vi "メイン.vi"() -> (2 "測定周期/ms":dbl, 3 "値転記用配列":T2[](array[typedef]))   [LabVIEW 2021] (continued)
                          n3920 = Add(x=6, y=w6513) -> (x+y=w6506:i32)
                          n3921 = Add(x=w6513, y=7) -> (x+y=w6504:i32)
                          n3922 = local read "csv作成表"() -> (w6500:string[][])
                          n3923 = Unbundle By Name(w6511) -> ("実測値(MAX)"=w6507:string, "実測値(MIN)"=w6508:string)
                          n3924 = Replace Array Subset(array=w6500, new element #1=w6507, index (row) #1=w6505, index (col) #1=w6506, new element #2=w6508, index (row) #2=w6505, index (col) #2=w6504) -> (w6502:string[][])
                          n3925 = Select(t=w6502, s=w6512, f=w6500) -> (s? t:f=w6503:string[][])
                          n3926 = local write "csv作成表"(w6503) -> ()
                        }
                        frame 5 {
                          w6523 = 2
                          # "B"
                          # "A"
                          # "csv作成の為表へクラスタ(実測値)書き込み"
                          # "⑤"
                          # "③"
                          # "④"
                          n3927 = local read "メインON/OFF_\n設定 6"() -> (w6534:T1)
                          n3928 = Unbundle By Name(w6534) -> ("使用ON/OFF"=w6530:bool)
                          n3929 = control-ref of="前回値転記用配列"() -> (w6528:refnum<vi>)
                          n3930 = local read "メイン設定_設定 6"() -> (w6535:T2)
                          n3931 = call "メイン_測定値配列_CSV転記サブ.vi"("メイン設定_設定入力"=w6535, "ループ反復数値入力"=w6532, "実測設定項目"=w6533, "使用ON/OFF"=w6530, "前回値転記用配列"=w6528) -> ("ループ反復数値出力"=w6531:i32, "メイン設定_設定出力"=w6529:T2)  [unwired: 5 in]
                          n3932 = local write "メイン設定_設定 6"(w6529) -> ()
                          n3933 = Add(x=7, y=w6531) -> (x+y=w6524:i32)
                          n3934 = Add(x=w6531, y=8) -> (x+y=w6522:i32)
                          n3935 = local read "csv作成表"() -> (w6518:string[][])
                          n3936 = Unbundle By Name(w6529) -> ("実測値(MAX)"=w6525:string, "実測値(MIN)"=w6526:string)
                          n3937 = Replace Array Subset(array=w6518, new element #1=w6525, index (row) #1=w6523, index (col) #1=w6524, new element #2=w6526, index (row) #2=w6523, index (col) #2=w6522) -> (w6520:string[][])
                          n3938 = Select(t=w6520, s=w6530, f=w6518) -> (s? t:f=w6521:string[][])
                          n3939 = local write "csv作成表"(w6521) -> ()
                        }
                        frame 6 {
                          w6541 = 2
                          # "B"
                          # "A"
                          # "csv作成の為表へクラスタ(実測値)書き込み"
                          # "⑤"
                          # "③"
                          # "④"
                          n3940 = local read "メインON/OFF_\n設定 7"() -> (w6552:T1)
                          n3941 = Unbundle By Name(w6552) -> ("使用ON/OFF"=w6548:bool)
                          n3942 = control-ref of="前回値転記用配列"() -> (w6546:refnum<vi>)
                          n3943 = local read "メイン設定_設定 7"() -> (w6553:T2)
                          n3944 = call "メイン_測定値配列_CSV転記サブ.vi"("メイン設定_設定入力"=w6553, "ループ反復数値入力"=w6550, "実測設定項目"=w6551, "使用ON/OFF"=w6548, "前回値転記用配列"=w6546) -> ("ループ反復数値出力"=w6549:i32, "メイン設定_設定出力"=w6547:T2)  [unwired: 5 in]
                          n3945 = local write "メイン設定_設定 7"(w6547) -> ()
                          n3946 = Add(x=8, y=w6549) -> (x+y=w6542:i32)
                          n3947 = Add(x=w6549, y=9) -> (x+y=w6540:i32)
                          n3948 = local read "csv作成表"() -> (w6536:string[][])
                          n3949 = Unbundle By Name(w6547) -> ("実測値(MAX)"=w6543:string, "実測値(MIN)"=w6544:string)
                          n3950 = Replace Array Subset(array=w6536, new element #1=w6543, index (row) #1=w6541, index (col) #1=w6542, new element #2=w6544, index (row) #2=w6541, index (col) #2=w6540) -> (w6538:string[][])
                          n3951 = Select(t=w6538, s=w6548, f=w6536) -> (s? t:f=w6539:string[][])
                          n3952 = local write "csv作成表"(w6539) -> ()
                        }
                        frame 7 {
                          w6559 = 2
                          # "B"
                          # "A"
                          # "csv作成の為表へクラスタ(実測値)書き込み"
                          # "⑤"
                          # "③"
                          # "④"
                          n3953 = local read "メインON/OFF_\n設定 8"() -> (w6570:T1)
                          n3954 = Unbundle By Name(w6570) -> ("使用ON/OFF"=w6566:bool)
                          n3955 = control-ref of="前回値転記用配列"() -> (w6564:refnum<vi>)
                          n3956 = local read "メイン設定_設定 8"() -> (w6571:T2)
                          n3957 = call "メイン_測定値配列_CSV転記サブ.vi"("メイン設定_設定入力"=w6571, "ループ反復数値入力"=w6568, "実測設定項目"=w6569, "使用ON/OFF"=w6566, "前回値転記用配列"=w6564) -> ("ループ反復数値出力"=w6567:i32, "メイン設定_設定出力"=w6565:T2)  [unwired: 5 in]
                          n3958 = local write "メイン設定_設定 8"(w6565) -> ()
                          n3959 = Add(x=9, y=w6567) -> (x+y=w6560:i32)
                          n3960 = Add(x=w6567, y=10) -> (x+y=w6558:i32)
                          n3961 = local read "csv作成表"() -> (w6554:string[][])
                          n3962 = Unbundle By Name(w6565) -> ("実測値(MAX)"=w6561:string, "実測値(MIN)"=w6562:string)
                          n3963 = Replace Array Subset(array=w6554, new element #1=w6561, index (row) #1=w6559, index (col) #1=w6560, new element #2=w6562, index (row) #2=w6559, index (col) #2=w6558) -> (w6556:string[][])
                          n3964 = Select(t=w6556, s=w6566, f=w6554) -> (s? t:f=w6557:string[][])
                          n3965 = local write "csv作成表"(w6557) -> ()
                        }
                        frame 8 {
                          w6577 = 2
                          # "B"
                          # "A"
                          # "csv作成の為表へクラスタ(実測値)書き込み"
                          # "⑤"
                          # "③"
                          # "④"
                          n3966 = local read "メインON/OFF_\n設定 9"() -> (w6588:T1)
                          n3967 = Unbundle By Name(w6588) -> ("使用ON/OFF"=w6584:bool)
                          n3968 = control-ref of="前回値転記用配列"() -> (w6582:refnum<vi>)
                          n3969 = local read "メイン設定_設定 9"() -> (w6589:T2)
                          n3970 = call "メイン_測定値配列_CSV転記サブ.vi"("メイン設定_設定入力"=w6589, "ループ反復数値入力"=w6586, "実測設定項目"=w6587, "使用ON/OFF"=w6584, "前回値転記用配列"=w6582) -> ("ループ反復数値出力"=w6585:i32, "メイン設定_設定出力"=w6583:T2)  [unwired: 5 in]
                          n3971 = local write "メイン設定_設定 9"(w6583) -> ()
                          n3972 = Add(x=10, y=w6585) -> (x+y=w6578:i32)
                          n3973 = Add(x=w6585, y=11) -> (x+y=w6576:i32)
                          n3974 = local read "csv作成表"() -> (w6572:string[][])
                          n3975 = Unbundle By Name(w6583) -> ("実測値(MAX)"=w6579:string, "実測値(MIN)"=w6580:string)
                          n3976 = Replace Array Subset(array=w6572, new element #1=w6579, index (row) #1=w6577, index (col) #1=w6578, new element #2=w6580, index (row) #2=w6577, index (col) #2=w6576) -> (w6574:string[][])
                          n3977 = Select(t=w6574, s=w6584, f=w6572) -> (s? t:f=w6575:string[][])
                          n3978 = local write "csv作成表"(w6575) -> ()
                        }
                        frame 9 {
                          w6595 = 2
                          # "B"
                          # "A"
                          # "csv作成の為表へクラスタ(実測値)書き込み"
                          # "⑤"
                          # "③"
                          # "④"
                          n3979 = local read "メインON/OFF_\n設定 10"() -> (w6606:T1)
                          n3980 = Unbundle By Name(w6606) -> ("使用ON/OFF"=w6602:bool)
                          n3981 = control-ref of="前回値転記用配列"() -> (w6600:refnum<vi>)
                          n3982 = local read "メイン設定_設定 10"() -> (w6607:T2)
                          n3983 = call "メイン_測定値配列_CSV転記サブ.vi"("メイン設定_設定入力"=w6607, "ループ反復数値入力"=w6604, "実測設定項目"=w6605, "使用ON/OFF"=w6602, "前回値転記用配列"=w6600) -> ("ループ反復数値出力"=w6603:i32, "メイン設定_設定出力"=w6601:T2)  [unwired: 5 in]
                          n3984 = local write "メイン設定_設定 10"(w6601) -> ()
                          n3985 = Add(x=11, y=w6603) -> (x+y=w6596:i32)
                          n3986 = Add(x=w6603, y=12) -> (x+y=w6594:i32)
                          n3987 = local read "csv作成表"() -> (w6590:string[][])
                          n3988 = Unbundle By Name(w6601) -> ("実測値(MAX)"=w6597:string, "実測値(MIN)"=w6598:string)
                          n3989 = Replace Array Subset(array=w6590, new element #1=w6597, index (row) #1=w6595, index (col) #1=w6596, new element #2=w6598, index (row) #2=w6595, index (col) #2=w6594) -> (w6592:string[][])
                          n3990 = Select(t=w6592, s=w6602, f=w6590) -> (s? t:f=w6593:string[][])
                          n3991 = local write "csv作成表"(w6593) -> ()
                        }
                        frame 10 {
                          w6613 = 2
                          # "B"
                          # "A"
                          # "csv作成の為表へクラスタ(実測値)書き込み"
                          # "⑤"
                          # "③"
                          # "④"
                          n3992 = local read "メインON/OFF_\n設定 11"() -> (w6624:T1)
                          n3993 = Unbundle By Name(w6624) -> ("使用ON/OFF"=w6620:bool)
                          n3994 = control-ref of="前回値転記用配列"() -> (w6618:refnum<vi>)
                          n3995 = local read "メイン設定_設定 11"() -> (w6625:T2)
                          n3996 = call "メイン_測定値配列_CSV転記サブ.vi"("メイン設定_設定入力"=w6625, "ループ反復数値入力"=w6622, "実測設定項目"=w6623, "使用ON/OFF"=w6620, "前回値転記用配列"=w6618) -> ("ループ反復数値出力"=w6621:i32, "メイン設定_設定出力"=w6619:T2)  [unwired: 5 in]
                          n3997 = local write "メイン設定_設定 11"(w6619) -> ()
                          n3998 = Add(x=12, y=w6621) -> (x+y=w6614:i32)
                          n3999 = Add(x=w6621, y=13) -> (x+y=w6612:i32)
                          n4000 = local read "csv作成表"() -> (w6608:string[][])
                          n4001 = Unbundle By Name(w6619) -> ("実測値(MAX)"=w6615:string, "実測値(MIN)"=w6616:string)
                          n4002 = Replace Array Subset(array=w6608, new element #1=w6615, index (row) #1=w6613, index (col) #1=w6614, new element #2=w6616, index (row) #2=w6613, index (col) #2=w6612) -> (w6610:string[][])
                          n4003 = Select(t=w6610, s=w6620, f=w6608) -> (s? t:f=w6611:string[][])
                          n4004 = local write "csv作成表"(w6611) -> ()
                        }
                        frame 11 {
                          w6631 = 2
                          # "B"
                          # "A"
                          # "csv作成の為表へクラスタ(実測値)書き込み"
                          # "⑤"
                          # "③"
                          # "④"
                          n4005 = local read "メインON/OFF_\n設定 12"() -> (w6642:T1)
                          n4006 = Unbundle By Name(w6642) -> ("使用ON/OFF"=w6638:bool)
                          n4007 = control-ref of="前回値転記用配列"() -> (w6636:refnum<vi>)
                          n4008 = local read "メイン設定_設定 12"() -> (w6643:T2)
                          n4009 = call "メイン_測定値配列_CSV転記サブ.vi"("メイン設定_設定入力"=w6643, "ループ反復数値入力"=w6640, "実測設定項目"=w6641, "使用ON/OFF"=w6638, "前回値転記用配列"=w6636) -> ("ループ反復数値出力"=w6639:i32, "メイン設定_設定出力"=w6637:T2)  [unwired: 5 in]
                          n4010 = local write "メイン設定_設定 12"(w6637) -> ()
                          n4011 = Add(x=13, y=w6639) -> (x+y=w6632:i32)
                          n4012 = Add(x=w6639, y=14) -> (x+y=w6630:i32)
                          n4013 = local read "csv作成表"() -> (w6626:string[][])
                          n4014 = Unbundle By Name(w6637) -> ("実測値(MAX)"=w6633:string, "実測値(MIN)"=w6634:string)
                          n4015 = Replace Array Subset(array=w6626, new element #1=w6633, index (row) #1=w6631, index (col) #1=w6632, new element #2=w6634, index (row) #2=w6631, index (col) #2=w6630) -> (w6628:string[][])
                          n4016 = Select(t=w6628, s=w6638, f=w6626) -> (s? t:f=w6629:string[][])
                          n4017 = local write "csv作成表"(w6629) -> ()
                        }
                      }
                    }
                  }
                }
                n4018 = local write "値転記用配列"(w6400) -> ()
                n4019 = flat-sequence {
                  tunnel: [w6415] -> w6401
                  tunnel: w6400 -> [w6415]
                  frame #0 {
                    w6410 = T9 {"Horizontal"=-51, "Vertical"=792} ("座標 11")
                    n4020 = control-ref of="このVI"() -> (w6414:refnum<vi>)
                    n4021 = property on="ペーン 2" class="Pane"("Origin"=w6410) -> ()  [unwired: 2 in, 2 out]
                    n4022 = property on="ペーン 2" class="Pane"("Origin"=w6410) -> ()  [unwired: 2 in, 2 out]
                    n4023 = control-ref of="このVI"() -> (w6412:refnum<vi>)
                    n4024 = Unbundle(w6410) -> ("Vertical"=w6413:i16)  [unwired: 1 out]
                    n4025 = Unbundle(w6410) -> ("Vertical"=w6411:i16)  [unwired: 1 out]
                    n4026 = call "メイン_装飾移動サブ.vi"("Y軸座標入力"=w6413, "VI入力"=w6414) -> ()  [unwired: 10 in]
                    n4027 = call "メイン_装飾枠移動サブ.vi"("Y軸座標入力"=w6411, "VI入力"=w6412) -> ()  [unwired: 10 in]
                  }
                }
              }
              frame #1 {
                w6646 = T8."Enabled" ("無効")
                # "⑪ボタンの無効解除"
                n4028 = for {
                  N: 12 -> [_]
                  tunnel: w6646 -> [w6648]
                  i -> [w6649]
                  n4029 = case shown="11" w6649 {
                    tunnel: w6648 -> [w6650 w6651 w6652 w6653 w6654 w6655 w6656 w6657 w6658 w6659 w6660 w6661]
                    frame 0, Default {
                      n4030 = property on="メイン測定ボタン_単発 1" class="Bool (指定)"("DisabledEnum"=w6650) -> ()  [unwired: 2 in, 2 out]
                      n4031 = property on="メイン測定ボタン_連続 1" class="Bool (指定)"("DisabledEnum"=w6650) -> ()  [unwired: 2 in, 2 out]
                    }
                    frame 1 {
                      n4032 = property on="メイン測定ボタン_単発 2" class="Bool (指定)"("DisabledEnum"=w6651) -> ()  [unwired: 2 in, 2 out]
                      n4033 = property on="メイン測定ボタン_連続 2" class="Bool (指定)"("DisabledEnum"=w6651) -> ()  [unwired: 2 in, 2 out]
                    }
                    frame 2 {
                      n4034 = property on="メイン測定ボタン_単発 3" class="Bool (指定)"("DisabledEnum"=w6652) -> ()  [unwired: 2 in, 2 out]
                      n4035 = property on="メイン測定ボタン_連続 3" class="Bool (指定)"("DisabledEnum"=w6652) -> ()  [unwired: 2 in, 2 out]
                    }
                    frame 3 {
                      n4036 = property on="メイン測定ボタン_単発 4" class="Bool (指定)"("DisabledEnum"=w6653) -> ()  [unwired: 2 in, 2 out]
                      n4037 = property on="メイン測定ボタン_連続 4" class="Bool (指定)"("DisabledEnum"=w6653) -> ()  [unwired: 2 in, 2 out]
                    }
                    frame 4 {
                      n4038 = property on="メイン測定ボタン_単発 5" class="Bool (指定)"("DisabledEnum"=w6654) -> ()  [unwired: 2 in, 2 out]
                      n4039 = property on="メイン測定ボタン_連続 5" class="Bool (指定)"("DisabledEnum"=w6654) -> ()  [unwired: 2 in, 2 out]
                    }
                    frame 5 {
                      n4040 = property on="メイン測定ボタン_連続 6" class="Bool (指定)"("DisabledEnum"=w6655) -> ()  [unwired: 2 in, 2 out]
                      n4041 = property on="メイン測定ボタン_単発 6" class="Bool (指定)"("DisabledEnum"=w6655) -> ()  [unwired: 2 in, 2 out]
                    }
                    frame 6 {
                      n4042 = property on="メイン測定ボタン_連続 7" class="Bool (指定)"("DisabledEnum"=w6656) -> ()  [unwired: 2 in, 2 out]
                      n4043 = property on="メイン測定ボタン_単発 7" class="Bool (指定)"("DisabledEnum"=w6656) -> ()  [unwired: 2 in, 2 out]
                    }
                    frame 7 {
                      n4044 = property on="メイン測定ボタン_単発 8" class="Bool (指定)"("DisabledEnum"=w6657) -> ()  [unwired: 2 in, 2 out]
                      n4045 = property on="メイン測定ボタン_連続 8" class="Bool (指定)"("DisabledEnum"=w6657) -> ()  [unwired: 2 in, 2 out]
                    }
                    frame 8 {
                      n4046 = property on="メイン測定ボタン_単発 9" class="Bool (指定)"("DisabledEnum"=w6658) -> ()  [unwired: 2 in, 2 out]
                      n4047 = property on="メイン測定ボタン_連続 9" class="Bool (指定)"("DisabledEnum"=w6658) -> ()  [unwired: 2 in, 2 out]
                    }
                    frame 9 {
                      n4048 = property on="メイン測定ボタン_単発 10" class="Bool (指定)"("DisabledEnum"=w6659) -> ()  [unwired: 2 in, 2 out]
                      n4049 = property on="メイン測定ボタン_連続 10" class="Bool (指定)"("DisabledEnum"=w6659) -> ()  [unwired: 2 in, 2 out]
                    }
                    frame 10 {
                      n4050 = property on="メイン測定ボタン_単発 11" class="Bool (指定)"("DisabledEnum"=w6660) -> ()  [unwired: 2 in, 2 out]
                      n4051 = property on="メイン測定ボタン_連続 11" class="Bool (指定)"("DisabledEnum"=w6660) -> ()  [unwired: 2 in, 2 out]
                    }
                    frame 11 {
                      n4052 = property on="メイン測定ボタン_連続 12" class="Bool (指定)"("DisabledEnum"=w6661) -> ()  [unwired: 2 in, 2 out]
                      n4053 = property on="メイン測定ボタン_単発 12" class="Bool (指定)"("DisabledEnum"=w6661) -> ()  [unwired: 2 in, 2 out]
                    }
                  }
                }
                n4054 = local write "測定新値\nリセット用 12"(TRUE) -> ()
                n4055 = property on="TOPページへ" class="Bool"("DisabledEnum"=w6646) -> ()  [unwired: 2 in, 2 out]
                n4056 = property on="保存して終了" class="Bool"("DisabledEnum"=w6646) -> ()  [unwired: 2 in, 2 out]
                n4057 = property on="保存せずに" class="Bool"("DisabledEnum"=w6646) -> ()  [unwired: 2 in, 2 out]
              }
            }
          }
          frame True {
          }
        }
      }
    }
    n4058 = Wait (ms)(milliseconds to wait=10) -> ()  [unwired: 1 out]
  }
  n4059 = while {
    tunnel: w1 -> [w6668]
    tunnel: [w6667] -> w9
    shift-right: [w6664] -> w8
    shift-left: w2 -> [w6666]
    stop <- w6665 stop-if-true
    # "メインページのボタン操作時の動作"
    n4060 = event shown="[15] \"メイン測定ボタン_連続 1\": 値変更" {
      selector: _ -> [_ _ _ _ _ _ _ _ _ _ _ _ _ _ _ _ _ _ _ _ _ _ _ _ _ _ _ _ _ _ _ _ _ _ _ _ _ _ _ _ _ _ _ _ _ _ _ _ _ _ _]
      dyn-events: _ -> [_ _ _ _ _ _ _ _ _ _ _ _ _ _ _ _ _ _ _ _ _ _ _ _ _ _ _ _ _ _ _ _ _ _ _ _ _ _ _ _ _ _ _ _ _ _ _ _ _ _ _]
      timeout: _ -> [_ _ _ _ _ _ _ _ _ _ _ _ _ _ _ _ _ _ _ _ _ _ _ _ _ _ _ _ _ _ _ _ _ _ _ _ _ _ _ _ _ _ _ _ _ _ _ _ _ _ _]
      tunnel: w6668 -> [w6673 w6676 w6681 w6686 w6691 w6696 w6701 w6706 w6711 w6716 w6721 w6726 w6731 w6736 w6741 w6752 w6791 w6830 w6869 w6908 w6947 w6986 w7025 w7064 w7103 w7142 w7181 w7223 w7334 w7445 w7556 w7667 w7778 w7889 w8000 w8111 w8222 w8333 w8444 w8543 w8546 w8549 w8552 w8555 w8558 w8561 w8564 w8567 w8570 w8573 w8576]
      tunnel: [_ _ _ w6685 w6690 w6695 w6700 w6705 w6710 w6715 w6720 w6725 w6730 w6735 w6740 w6751 w6790 w6829 w6868 w6907 w6946 w6985 w7024 w7063 w7102 w7141 w7180 w7224 w7335 w7446 w7557 w7668 w7779 w7890 w8001 w8112 w8223 w8334 w8445 _ _ _ _ _ _ _ _ _ _ _ _] -> w6667
      tunnel: w6666 -> [w6671 w6674 w6680 w6683 w6688 w6693 w6698 w6703 w6708 w6713 w6718 w6723 w6728 w6733 w6738 w6749 w6788 w6827 w6866 w6905 w6944 w6983 w7022 w7061 w7100 w7139 w7178 w7221 w7332 w7443 w7554 w7665 w7776 w7887 w7998 w8109 w8220 w8331 w8442 w8542 w8545 w8548 w8551 w8554 w8557 w8560 w8563 w8566 w8569 w8572 w8575]
      tunnel: [w6672 w6675 w6678 w6684 w6689 w6694 w6699 w6704 w6709 w6714 w6719 w6724 w6729 w6734 w6739 w6750 w6789 w6828 w6867 w6906 w6945 w6984 w7023 w7062 w7101 w7140 w7179 w7222 w7333 w7444 w7555 w7666 w7777 w7888 w7999 w8110 w8221 w8332 w8443 _ _ _ _ _ _ _ _ _ _ _ _] -> w6664
      tunnel: [TRUE _ _ _ _ _ _ _ _ _ _ _ _ _ _ _ _ _ _ _ _ _ _ _ _ _ _ _ _ _ _ _ _ _ _ _ _ _ _ _ _ _ _ _ _ _ _ _ _ _ _] -> w6665
      tunnel: T8."Disabled" ("無効") -> [_ _ _ _ _ _ _ _ _ _ _ _ _ _ _ w6748 w6787 w6826 w6865 w6904 w6943 w6982 w7021 w7060 w7099 w7138 w7176 _ _ _ _ _ _ _ _ _ _ _ _ _ _ _ _ _ _ _ _ _ _ _ _]
      event "TOPページへ": Value Change {
        n4061 = event-data() -> ()  [unwired: 1 in, 6 out]
        n4062 = Enqueue Element(queue=w6673, element="TOPページへ", error in (no error)=w6671) -> (error out=w6672:errorcluster)  [unwired: 1 in, 2 out]
      }
      event "保存せずに": Value Change {
        # "メインページの保存せずに終了ボタンが押された時に動作"
        n4063 = event-data() -> ()  [unwired: 1 in, 1 out]
        n4064 = Enqueue Element(queue=w6676, element="保存せず", error in (no error)=w6674) -> (error out=w6675:errorcluster)  [unwired: 1 in, 2 out]
      }
      event "保存して終了": Value Change {
        n4065 = event-data() -> ()  [unwired: 1 in, 1 out]
        n4066 = Enqueue Element(queue=w6681, element="保存して終了", error in (no error)=w6680) -> (error out=w6678:errorcluster)  [unwired: 1 in, 2 out]
      }
      event Value Change {
        n4067 = event-data() -> ()  [unwired: 1 in, 6 out]
        n4068 = Enqueue Element(queue=w6686, element="値1クリア", error in (no error)=w6683) -> (queue out=w6685:refnum<queue>, error out=w6684:errorcluster)  [unwired: 1 in, 1 out]
      }
      event Value Change {
        # "①"
        # "複製時に変更する項目\n①キュー"
        n4069 = event-data() -> ()  [unwired: 1 in, 6 out]
        n4070 = Enqueue Element(queue=w6691, element="値2クリア", error in (no error)=w6688) -> (queue out=w6690:refnum<queue>, error out=w6689:errorcluster)  [unwired: 1 in, 1 out]
      }
      event Value Change {
        # "①"
        # "複製時に変更する項目\n①キュー"
        n4071 = event-data() -> ()  [unwired: 1 in, 6 out]
        n4072 = Enqueue Element(queue=w6696, element="値3クリア", error in (no error)=w6693) -> (queue out=w6695:refnum<queue>, error out=w6694:errorcluster)  [unwired: 1 in, 1 out]
      }
      event Value Change {
        # "①"
        # "複製時に変更する項目\n①キュー"
        n4073 = event-data() -> ()  [unwired: 1 in, 6 out]
        n4074 = Enqueue Element(queue=w6701, element="値4クリア", error in (no error)=w6698) -> (queue out=w6700:refnum<queue>, error out=w6699:errorcluster)  [unwired: 1 in, 1 out]
      }
      event Value Change {
        # "①"
        # "複製時に変更する項目\n①キュー"
        n4075 = event-data() -> ()  [unwired: 1 in, 6 out]
        n4076 = Enqueue Element(queue=w6706, element="値5クリア", error in (no error)=w6703) -> (queue out=w6705:refnum<queue>, error out=w6704:errorcluster)  [unwired: 1 in, 1 out]
      }
      event Value Change {
        # "①"
        # "複製時に変更する項目\n①キュー"
        n4077 = event-data() -> ()  [unwired: 1 in, 6 out]
        n4078 = Enqueue Element(queue=w6711, element="値6クリア", error in (no error)=w6708) -> (queue out=w6710:refnum<queue>, error out=w6709:errorcluster)  [unwired: 1 in, 1 out]
      }
      event Value Change {
        # "①"
        # "複製時に変更する項目\n①キュー"
        n4079 = event-data() -> ()  [unwired: 1 in, 6 out]
        n4080 = Enqueue Element(queue=w6716, element="値7クリア", error in (no error)=w6713) -> (queue out=w6715:refnum<queue>, error out=w6714:errorcluster)  [unwired: 1 in, 1 out]
      }
      event Value Change {
        # "①"
        # "複製時に変更する項目\n①キュー"
        n4081 = event-data() -> ()  [unwired: 1 in, 6 out]
        n4082 = Enqueue Element(queue=w6721, element="値8クリア", error in (no error)=w6718) -> (queue out=w6720:refnum<queue>, error out=w6719:errorcluster)  [unwired: 1 in, 1 out]
      }
      event Value Change {
        # "①"
        # "複製時に変更する項目\n①キュー"
        n4083 = event-data() -> ()  [unwired: 1 in, 6 out]
        n4084 = Enqueue Element(queue=w6726, element="値9クリア", error in (no error)=w6723) -> (queue out=w6725:refnum<queue>, error out=w6724:errorcluster)  [unwired: 1 in, 1 out]
      }
      event Value Change {
        # "①"
        # "複製時に変更する項目\n①キュー"
        n4085 = event-data() -> ()  [unwired: 1 in, 6 out]
        n4086 = Enqueue Element(queue=w6731, element="値10クリア", error in (no error)=w6728) -> (queue out=w6730:refnum<queue>, error out=w6729:errorcluster)  [unwired: 1 in, 1 out]
      }
      event Value Change {
        # "①"
        # "複製時に変更する項目\n①キュー"
        n4087 = event-data() -> ()  [unwired: 1 in, 6 out]
        n4088 = Enqueue Element(queue=w6736, element="値11クリア", error in (no error)=w6733) -> (queue out=w6735:refnum<queue>, error out=w6734:errorcluster)  [unwired: 1 in, 1 out]
      }
      event Value Change {
        # "①"
        # "複製時に変更する項目\n①キュー"
        n4089 = event-data() -> ()  [unwired: 1 in, 6 out]
        n4090 = Enqueue Element(queue=w6741, element="値12クリア", error in (no error)=w6738) -> (queue out=w6740:refnum<queue>, error out=w6739:errorcluster)  [unwired: 1 in, 1 out]
      }
      event Value Change {
        w6742 = 12
        # "※複製時\n①ブールボタン\n測定旧値\nが複製されているか確認\n②測定新値リセット用の作成\n対象の以外をリセットする\n③対象の連続ボタン以外複製する"
        # "②　例ケースが”メイン測定ボタン_連続2”の場合、\n測定新値リセット用2以外をリセットする"
        # "①"
        n4091 = event-data() -> ("OldVal"=w6745:T6)  [unwired: 1 in, 2 out]
        "測定旧値 1" <- w6745
        n4092 = Enqueue Element(queue=w6752, element="測定1", error in (no error)=w6749) -> (queue out=w6751:refnum<queue>, error out=w6750:errorcluster)  [unwired: 1 in, 1 out]
        n4093 = Select(t=TRUE, s=w6745, f=FALSE) -> (s? t:f=w6744:bool)
        n4094 = global write "測定キャンセルボタン.vi" "グローバル_測定キャンセルボタン"(w6744) -> ()
        n4095 = local write "G_メイン測定キャンセルボタン"(w6744) -> ()
        n4096 = for {
          N: w6742 -> [_]
          tunnel: FALSE -> [w6754]
          i -> [w6755]
          n4097 = case shown="0, デフォルト" w6755 {
            tunnel: w6754 -> [_ w6756 w6757 w6758 w6759 w6760 w6761 w6762 w6763 w6764 w6765 w6766]
            frame 0, Default {
            }
            frame 1 {
              n4098 = local write "測定新値\nリセット用 2"(w6756) -> ()
            }
            frame 2 {
              n4099 = local write "測定新値\nリセット用 3"(w6757) -> ()
            }
            frame 3 {
              n4100 = local write "測定新値\nリセット用 4"(w6758) -> ()
            }
            frame 4 {
              n4101 = local write "測定新値\nリセット用 5"(w6759) -> ()
            }
            frame 5 {
              n4102 = local write "測定新値\nリセット用 6"(w6760) -> ()
            }
            frame 6 {
              n4103 = local write "測定新値\nリセット用 7"(w6761) -> ()
            }
            frame 7 {
              n4104 = local write "測定新値\nリセット用 8"(w6762) -> ()
            }
            frame 8 {
              n4105 = local write "測定新値\nリセット用 9"(w6763) -> ()
            }
            frame 9 {
              n4106 = local write "測定新値\nリセット用 10"(w6764) -> ()
            }
            frame 10 {
              n4107 = local write "測定新値\nリセット用 11"(w6765) -> ()
            }
            frame 11 {
              n4108 = local write "測定新値\nリセット用 12"(w6766) -> ()
            }
          }
        }
        n4109 = for {
          N: w6742 -> [_]
          tunnel: w6748 -> [w6767]
          i -> [w6768]
          n4110 = case shown="0, デフォルト" w6768 {
            tunnel: w6767 -> [w6769 w6770 w6771 w6772 w6773 w6774 w6775 w6776 w6777 w6778 w6779 w6780]
            frame 0, Default {
              n4111 = property on="メイン測定ボタン_単発 1" class="Bool (指定)"("DisabledEnum"=w6769) -> ()  [unwired: 2 in, 2 out]
            }
            frame 1 {
              n4112 = property on="メイン測定ボタン_単発 2" class="Bool (指定)"("DisabledEnum"=w6770) -> ()  [unwired: 2 in, 2 out]
              n4113 = property on="メイン測定ボタン_連続 2" class="Bool (指定)"("DisabledEnum"=w6770) -> ()  [unwired: 2 in, 2 out]
            }
            frame 2 {
              n4114 = property on="メイン測定ボタン_単発 3" class="Bool (指定)"("DisabledEnum"=w6771) -> ()  [unwired: 2 in, 2 out]
              n4115 = property on="メイン測定ボタン_連続 3" class="Bool (指定)"("DisabledEnum"=w6771) -> ()  [unwired: 2 in, 2 out]
            }
            frame 3 {
              n4116 = property on="メイン測定ボタン_単発 4" class="Bool (指定)"("DisabledEnum"=w6772) -> ()  [unwired: 2 in, 2 out]
              n4117 = property on="メイン測定ボタン_連続 4" class="Bool (指定)"("DisabledEnum"=w6772) -> ()  [unwired: 2 in, 2 out]
            }
            frame 4 {
              n4118 = property on="メイン測定ボタン_単発 5" class="Bool (指定)"("DisabledEnum"=w6773) -> ()  [unwired: 2 in, 2 out]
              n4119 = property on="メイン測定ボタン_連続 5" class="Bool (指定)"("DisabledEnum"=w6773) -> ()  [unwired: 2 in, 2 out]
            }
            frame 5 {
              n4120 = property on="メイン測定ボタン_連続 6" class="Bool (指定)"("DisabledEnum"=w6774) -> ()  [unwired: 2 in, 2 out]
              n4121 = property on="メイン測定ボタン_単発 6" class="Bool (指定)"("DisabledEnum"=w6774) -> ()  [unwired: 2 in, 2 out]
            }
            frame 6 {
              n4122 = property on="メイン測定ボタン_連続 7" class="Bool (指定)"("DisabledEnum"=w6775) -> ()  [unwired: 2 in, 2 out]
              n4123 = property on="メイン測定ボタン_単発 7" class="Bool (指定)"("DisabledEnum"=w6775) -> ()  [unwired: 2 in, 2 out]
            }
            frame 7 {
              n4124 = property on="メイン測定ボタン_単発 8" class="Bool (指定)"("DisabledEnum"=w6776) -> ()  [unwired: 2 in, 2 out]
              n4125 = property on="メイン測定ボタン_連続 8" class="Bool (指定)"("DisabledEnum"=w6776) -> ()  [unwired: 2 in, 2 out]
            }
            frame 8 {
              n4126 = property on="メイン測定ボタン_単発 9" class="Bool (指定)"("DisabledEnum"=w6777) -> ()  [unwired: 2 in, 2 out]
              n4127 = property on="メイン測定ボタン_連続 9" class="Bool (指定)"("DisabledEnum"=w6777) -> ()  [unwired: 2 in, 2 out]
            }
            frame 9 {
              n4128 = property on="メイン測定ボタン_単発 10" class="Bool (指定)"("DisabledEnum"=w6778) -> ()  [unwired: 2 in, 2 out]
              n4129 = property on="メイン測定ボタン_連続 10" class="Bool (指定)"("DisabledEnum"=w6778) -> ()  [unwired: 2 in, 2 out]
            }
            frame 10 {
              n4130 = property on="メイン測定ボタン_単発 11" class="Bool (指定)"("DisabledEnum"=w6779) -> ()  [unwired: 2 in, 2 out]
              n4131 = property on="メイン測定ボタン_連続 11" class="Bool (指定)"("DisabledEnum"=w6779) -> ()  [unwired: 2 in, 2 out]
            }
            frame 11 {
              n4132 = property on="メイン測定ボタン_連続 12" class="Bool (指定)"("DisabledEnum"=w6780) -> ()  [unwired: 2 in, 2 out]
              n4133 = property on="メイン測定ボタン_単発 12" class="Bool (指定)"("DisabledEnum"=w6780) -> ()  [unwired: 2 in, 2 out]
            }
          }
        }
        n4134 = property on="TOPページへ" class="Bool"("DisabledEnum"=w6748) -> ()  [unwired: 2 in, 2 out]
        n4135 = property on="保存して終了" class="Bool"("DisabledEnum"=w6748) -> ()  [unwired: 2 in, 2 out]
        n4136 = property on="保存せずに" class="Bool"("DisabledEnum"=w6748) -> ()  [unwired: 2 in, 2 out]
      }
      event Value Change {
        w6781 = 12
        # "※複製時\n①ブールボタン\n測定旧値\nが複製されているか確認\n②測定新値リセット用の作成\n対象の以外をリセットする\n③\nキュー\n④対象の連続ボタン以外複製する"
        # "④ボタン操作時の他のボタン操作無効"
        # "③"
        # "旧値(ボタンが押される前と後)の値でグローバル_測定キャンセルボタンの\nTrue/Falseの切り替えを行う"
        # "②　例ケースが”メイン測定ボタン_連続2”の場合、\n測定新値リセット用2以外をリセットする"
        # "①"
        n4137 = event-data() -> ("OldVal"=w6783:T6)  [unwired: 1 in, 2 out]
        "測定旧値 2" <- w6783
        n4138 = Enqueue Element(queue=w6791, element="測定2", error in (no error)=w6788) -> (queue out=w6790:refnum<queue>, error out=w6789:errorcluster)  [unwired: 1 in, 1 out]
        n4139 = Select(t=TRUE, s=w6783, f=FALSE) -> (s? t:f=w6786:bool)
        n4140 = global write "測定キャンセルボタン.vi" "グローバル_測定キャンセルボタン"(w6786) -> ()
        n4141 = local write "G_メイン測定キャンセルボタン"(w6786) -> ()
        n4142 = for {
          N: w6781 -> [_]
          tunnel: FALSE -> [w6793]
          i -> [w6794]
          n4143 = case shown="1" w6794 {
            tunnel: w6793 -> [w6795 _ w6796 w6797 w6798 w6799 w6800 w6801 w6802 w6803 w6804 w6805]
            frame 0, Default {
              n4144 = local write "測定新値\nリセット用 1"(w6795) -> ()
            }
            frame 1 {
            }
            frame 2 {
              n4145 = local write "測定新値\nリセット用 3"(w6796) -> ()
            }
            frame 3 {
              n4146 = local write "測定新値\nリセット用 4"(w6797) -> ()
            }
            frame 4 {
              n4147 = local write "測定新値\nリセット用 5"(w6798) -> ()
            }
            frame 5 {
              n4148 = local write "測定新値\nリセット用 6"(w6799) -> ()
            }
            frame 6 {
              n4149 = local write "測定新値\nリセット用 7"(w6800) -> ()
            }
            frame 7 {
              n4150 = local write "測定新値\nリセット用 8"(w6801) -> ()
            }
            frame 8 {
              n4151 = local write "測定新値\nリセット用 9"(w6802) -> ()
            }
            frame 9 {
              n4152 = local write "測定新値\nリセット用 10"(w6803) -> ()
            }
            frame 10 {
              n4153 = local write "測定新値\nリセット用 11"(w6804) -> ()
            }
            frame 11 {
              n4154 = local write "測定新値\nリセット用 12"(w6805) -> ()
            }
          }
        }
        n4155 = for {
          N: w6781 -> [_]
          tunnel: w6787 -> [w6806]
          i -> [w6807]
          n4156 = case shown="11" w6807 {
            tunnel: w6806 -> [w6808 w6809 w6810 w6811 w6812 w6813 w6814 w6815 w6816 w6817 w6818 w6819]
            frame 0, Default {
              n4157 = property on="メイン測定ボタン_単発 1" class="Bool (指定)"("DisabledEnum"=w6808) -> ()  [unwired: 2 in, 2 out]
              n4158 = property on="メイン測定ボタン_連続 1" class="Bool (指定)"("DisabledEnum"=w6808) -> ()  [unwired: 2 in, 2 out]
            }
            frame 1 {
              n4159 = property on="メイン測定ボタン_単発 2" class="Bool (指定)"("DisabledEnum"=w6809) -> ()  [unwired: 2 in, 2 out]
            }
            frame 2 {
              n4160 = property on="メイン測定ボタン_単発 3" class="Bool (指定)"("DisabledEnum"=w6810) -> ()  [unwired: 2 in, 2 out]
              n4161 = property on="メイン測定ボタン_連続 3" class="Bool (指定)"("DisabledEnum"=w6810) -> ()  [unwired: 2 in, 2 out]
            }
            frame 3 {
              n4162 = property on="メイン測定ボタン_単発 4" class="Bool (指定)"("DisabledEnum"=w6811) -> ()  [unwired: 2 in, 2 out]
              n4163 = property on="メイン測定ボタン_連続 4" class="Bool (指定)"("DisabledEnum"=w6811) -> ()  [unwired: 2 in, 2 out]
            }
            frame 4 {
              n4164 = property on="メイン測定ボタン_単発 5" class="Bool (指定)"("DisabledEnum"=w6812) -> ()  [unwired: 2 in, 2 out]
              n4165 = property on="メイン測定ボタン_連続 5" class="Bool (指定)"("DisabledEnum"=w6812) -> ()  [unwired: 2 in, 2 out]
            }
            frame 5 {
              n4166 = property on="メイン測定ボタン_連続 6" class="Bool (指定)"("DisabledEnum"=w6813) -> ()  [unwired: 2 in, 2 out]
              n4167 = property on="メイン測定ボタン_単発 6" class="Bool (指定)"("DisabledEnum"=w6813) -> ()  [unwired: 2 in, 2 out]
            }
            frame 6 {
              n4168 = property on="メイン測定ボタン_連続 7" class="Bool (指定)"("DisabledEnum"=w6814) -> ()  [unwired: 2 in, 2 out]
              n4169 = property on="メイン測定ボタン_単発 7" class="Bool (指定)"("DisabledEnum"=w6814) -> ()  [unwired: 2 in, 2 out]
            }
            frame 7 {
              n4170 = property on="メイン測定ボタン_単発 8" class="Bool (指定)"("DisabledEnum"=w6815) -> ()  [unwired: 2 in, 2 out]
              n4171 = property on="メイン測定ボタン_連続 8" class="Bool (指定)"("DisabledEnum"=w6815) -> ()  [unwired: 2 in, 2 out]
            }
            frame 8 {
              n4172 = property on="メイン測定ボタン_単発 9" class="Bool (指定)"("DisabledEnum"=w6816) -> ()  [unwired: 2 in, 2 out]
              n4173 = property on="メイン測定ボタン_連続 9" class="Bool (指定)"("DisabledEnum"=w6816) -> ()  [unwired: 2 in, 2 out]
            }
            frame 9 {
              n4174 = property on="メイン測定ボタン_単発 10" class="Bool (指定)"("DisabledEnum"=w6817) -> ()  [unwired: 2 in, 2 out]
              n4175 = property on="メイン測定ボタン_連続 10" class="Bool (指定)"("DisabledEnum"=w6817) -> ()  [unwired: 2 in, 2 out]
            }
            frame 10 {
              n4176 = property on="メイン測定ボタン_単発 11" class="Bool (指定)"("DisabledEnum"=w6818) -> ()  [unwired: 2 in, 2 out]
              n4177 = property on="メイン測定ボタン_連続 11" class="Bool (指定)"("DisabledEnum"=w6818) -> ()  [unwired: 2 in, 2 out]
            }
            frame 11 {
              n4178 = property on="メイン測定ボタン_連続 12" class="Bool (指定)"("DisabledEnum"=w6819) -> ()  [unwired: 2 in, 2 out]
              n4179 = property on="メイン測定ボタン_単発 12" class="Bool (指定)"("DisabledEnum"=w6819) -> ()  [unwired: 2 in, 2 out]
            }
          }
        }
        n4180 = property on="TOPページへ" class="Bool"("DisabledEnum"=w6787) -> ()  [unwired: 2 in, 2 out]
        n4181 = property on="保存して終了" class="Bool"("DisabledEnum"=w6787) -> ()  [unwired: 2 in, 2 out]
        n4182 = property on="保存せずに" class="Bool"("DisabledEnum"=w6787) -> ()  [unwired: 2 in, 2 out]
      }
      event Value Change {
        w6820 = 12
        # "④ボタン操作時の他のボタン操作無効"
        # "※複製時\n①ブールボタン\n測定旧値\nが複製されているか確認\n②測定新値リセット用の作成\n対象の以外をリセットする\n③\nキュー\n④対象の連続ボタン以外複製する"
        # "③"
        # "旧値(ボタンが押される前と後)の値でグローバル_測定キャンセルボタンの\nTrue/Falseの切り替えを行う"
        # "②　例ケースが”メイン測定ボタン_連続2”の場合、\n測定新値リセット用2以外をリセットする"
        # "①"
        n4183 = event-data() -> ("OldVal"=w6822:T6)  [unwired: 1 in, 2 out]
        "測定旧値 3" <- w6822
        n4184 = Enqueue Element(queue=w6830, element="測定3", error in (no error)=w6827) -> (queue out=w6829:refnum<queue>, error out=w6828:errorcluster)  [unwired: 1 in, 1 out]
        n4185 = Select(t=TRUE, s=w6822, f=FALSE) -> (s? t:f=w6825:bool)
        n4186 = global write "測定キャンセルボタン.vi" "グローバル_測定キャンセルボタン"(w6825) -> ()
        n4187 = local write "G_メイン測定キャンセルボタン"(w6825) -> ()
        n4188 = for {
          N: w6820 -> [_]
          tunnel: FALSE -> [w6832]
          i -> [w6833]
          n4189 = case shown="2" w6833 {
            tunnel: w6832 -> [w6834 w6835 _ w6836 w6837 w6838 w6839 w6840 w6841 w6842 w6843 w6844]
            frame 0, Default {
              n4190 = local write "測定新値\nリセット用 1"(w6834) -> ()
            }
            frame 1 {
              n4191 = local write "測定新値\nリセット用 2"(w6835) -> ()
            }
            frame 2 {
            }
            frame 3 {
              n4192 = local write "測定新値\nリセット用 4"(w6836) -> ()
            }
            frame 4 {
              n4193 = local write "測定新値\nリセット用 5"(w6837) -> ()
            }
            frame 5 {
              n4194 = local write "測定新値\nリセット用 6"(w6838) -> ()
            }
            frame 6 {
              n4195 = local write "測定新値\nリセット用 7"(w6839) -> ()
            }
            frame 7 {
              n4196 = local write "測定新値\nリセット用 8"(w6840) -> ()
            }
            frame 8 {
              n4197 = local write "測定新値\nリセット用 9"(w6841) -> ()
            }
            frame 9 {
              n4198 = local write "測定新値\nリセット用 10"(w6842) -> ()
            }
            frame 10 {
              n4199 = local write "測定新値\nリセット用 11"(w6843) -> ()
            }
            frame 11 {
              n4200 = local write "測定新値\nリセット用 12"(w6844) -> ()
            }
          }
        }
        n4201 = for {
          N: w6820 -> [_]
          tunnel: w6826 -> [w6845]
          i -> [w6846]
          n4202 = case shown="11" w6846 {
            tunnel: w6845 -> [w6847 w6848 w6849 w6850 w6851 w6852 w6853 w6854 w6855 w6856 w6857 w6858]
            frame 0, Default {
              n4203 = property on="メイン測定ボタン_単発 1" class="Bool (指定)"("DisabledEnum"=w6847) -> ()  [unwired: 2 in, 2 out]
              n4204 = property on="メイン測定ボタン_連続 1" class="Bool (指定)"("DisabledEnum"=w6847) -> ()  [unwired: 2 in, 2 out]
            }
            frame 1 {
              n4205 = property on="メイン測定ボタン_単発 2" class="Bool (指定)"("DisabledEnum"=w6848) -> ()  [unwired: 2 in, 2 out]
              n4206 = property on="メイン測定ボタン_連続 2" class="Bool (指定)"("DisabledEnum"=w6848) -> ()  [unwired: 2 in, 2 out]
            }
            frame 2 {
              n4207 = property on="メイン測定ボタン_単発 3" class="Bool (指定)"("DisabledEnum"=w6849) -> ()  [unwired: 2 in, 2 out]
            }
            frame 3 {
              n4208 = property on="メイン測定ボタン_単発 4" class="Bool (指定)"("DisabledEnum"=w6850) -> ()  [unwired: 2 in, 2 out]
              n4209 = property on="メイン測定ボタン_連続 4" class="Bool (指定)"("DisabledEnum"=w6850) -> ()  [unwired: 2 in, 2 out]
            }
            frame 4 {
              n4210 = property on="メイン測定ボタン_単発 5" class="Bool (指定)"("DisabledEnum"=w6851) -> ()  [unwired: 2 in, 2 out]
              n4211 = property on="メイン測定ボタン_連続 5" class="Bool (指定)"("DisabledEnum"=w6851) -> ()  [unwired: 2 in, 2 out]
            }
            frame 5 {
              n4212 = property on="メイン測定ボタン_連続 6" class="Bool (指定)"("DisabledEnum"=w6852) -> ()  [unwired: 2 in, 2 out]
              n4213 = property on="メイン測定ボタン_単発 6" class="Bool (指定)"("DisabledEnum"=w6852) -> ()  [unwired: 2 in, 2 out]
            }
            frame 6 {
              n4214 = property on="メイン測定ボタン_連続 7" class="Bool (指定)"("DisabledEnum"=w6853) -> ()  [unwired: 2 in, 2 out]
              n4215 = property on="メイン測定ボタン_単発 7" class="Bool (指定)"("DisabledEnum"=w6853) -> ()  [unwired: 2 in, 2 out]
            }
            frame 7 {
              n4216 = property on="メイン測定ボタン_単発 8" class="Bool (指定)"("DisabledEnum"=w6854) -> ()  [unwired: 2 in, 2 out]
              n4217 = property on="メイン測定ボタン_連続 8" class="Bool (指定)"("DisabledEnum"=w6854) -> ()  [unwired: 2 in, 2 out]
            }
            frame 8 {
              n4218 = property on="メイン測定ボタン_単発 9" class="Bool (指定)"("DisabledEnum"=w6855) -> ()  [unwired: 2 in, 2 out]
              n4219 = property on="メイン測定ボタン_連続 9" class="Bool (指定)"("DisabledEnum"=w6855) -> ()  [unwired: 2 in, 2 out]
            }
            frame 9 {
              n4220 = property on="メイン測定ボタン_単発 10" class="Bool (指定)"("DisabledEnum"=w6856) -> ()  [unwired: 2 in, 2 out]
              n4221 = property on="メイン測定ボタン_連続 10" class="Bool (指定)"("DisabledEnum"=w6856) -> ()  [unwired: 2 in, 2 out]
            }
            frame 10 {
              n4222 = property on="メイン測定ボタン_単発 11" class="Bool (指定)"("DisabledEnum"=w6857) -> ()  [unwired: 2 in, 2 out]
              n4223 = property on="メイン測定ボタン_連続 11" class="Bool (指定)"("DisabledEnum"=w6857) -> ()  [unwired: 2 in, 2 out]
            }
            frame 11 {
              n4224 = property on="メイン測定ボタン_連続 12" class="Bool (指定)"("DisabledEnum"=w6858) -> ()  [unwired: 2 in, 2 out]
              n4225 = property on="メイン測定ボタン_単発 12" class="Bool (指定)"("DisabledEnum"=w6858) -> ()  [unwired: 2 in, 2 out]
            }
          }
        }
        n4226 = property on="TOPページへ" class="Bool"("DisabledEnum"=w6826) -> ()  [unwired: 2 in, 2 out]
        n4227 = property on="保存して終了" class="Bool"("DisabledEnum"=w6826) -> ()  [unwired: 2 in, 2 out]
        n4228 = property on="保存せずに" class="Bool"("DisabledEnum"=w6826) -> ()  [unwired: 2 in, 2 out]
      }
      event Value Change {
        w6859 = 12
        # "④ボタン操作時の他のボタン操作無効"
        # "※複製時\n①ブールボタン\n測定旧値\nが複製されているか確認\n②測定新値リセット用の作成\n対象の以外をリセットする\n③\nキュー\n④対象の連続ボタン以外複製する"
        # "③"
        # "旧値(ボタンが押される前と後)の値でグローバル_測定キャンセルボタンの\nTrue/Falseの切り替えを行う"
        # "②　例ケースが”メイン測定ボタン_連続2”の場合、\n測定新値リセット用2以外をリセットする"
        # "①"
        n4229 = event-data() -> ("OldVal"=w6861:T6)  [unwired: 1 in, 2 out]
        "測定旧値 4" <- w6861
        n4230 = Enqueue Element(queue=w6869, element="測定4", error in (no error)=w6866) -> (queue out=w6868:refnum<queue>, error out=w6867:errorcluster)  [unwired: 1 in, 1 out]
        n4231 = Select(t=TRUE, s=w6861, f=FALSE) -> (s? t:f=w6864:bool)
        n4232 = global write "測定キャンセルボタン.vi" "グローバル_測定キャンセルボタン"(w6864) -> ()
        n4233 = local write "G_メイン測定キャンセルボタン"(w6864) -> ()
        n4234 = for {
          N: w6859 -> [_]
          tunnel: FALSE -> [w6871]
          i -> [w6872]
          n4235 = case shown="3" w6872 {
            tunnel: w6871 -> [w6873 w6874 w6875 _ w6876 w6877 w6878 w6879 w6880 w6881 w6882 w6883]
            frame 0, Default {
              n4236 = local write "測定新値\nリセット用 1"(w6873) -> ()
            }
            frame 1 {
              n4237 = local write "測定新値\nリセット用 2"(w6874) -> ()
            }
            frame 2 {
              n4238 = local write "測定新値\nリセット用 3"(w6875) -> ()
            }
            frame 3 {
            }
            frame 4 {
              n4239 = local write "測定新値\nリセット用 5"(w6876) -> ()
            }
            frame 5 {
              n4240 = local write "測定新値\nリセット用 6"(w6877) -> ()
            }
            frame 6 {
              n4241 = local write "測定新値\nリセット用 7"(w6878) -> ()
            }
            frame 7 {
              n4242 = local write "測定新値\nリセット用 8"(w6879) -> ()
            }
            frame 8 {
              n4243 = local write "測定新値\nリセット用 9"(w6880) -> ()
            }
            frame 9 {
              n4244 = local write "測定新値\nリセット用 10"(w6881) -> ()
            }
            frame 10 {
              n4245 = local write "測定新値\nリセット用 11"(w6882) -> ()
            }
            frame 11 {
              n4246 = local write "測定新値\nリセット用 12"(w6883) -> ()
            }
          }
        }
        n4247 = for {
          N: w6859 -> [_]
          tunnel: w6865 -> [w6884]
          i -> [w6885]
          n4248 = case shown="11" w6885 {
            tunnel: w6884 -> [w6886 w6887 w6888 w6889 w6890 w6891 w6892 w6893 w6894 w6895 w6896 w6897]
            frame 0, Default {
              n4249 = property on="メイン測定ボタン_単発 1" class="Bool (指定)"("DisabledEnum"=w6886) -> ()  [unwired: 2 in, 2 out]
              n4250 = property on="メイン測定ボタン_連続 1" class="Bool (指定)"("DisabledEnum"=w6886) -> ()  [unwired: 2 in, 2 out]
            }
            frame 1 {
              n4251 = property on="メイン測定ボタン_単発 2" class="Bool (指定)"("DisabledEnum"=w6887) -> ()  [unwired: 2 in, 2 out]
              n4252 = property on="メイン測定ボタン_連続 2" class="Bool (指定)"("DisabledEnum"=w6887) -> ()  [unwired: 2 in, 2 out]
            }
            frame 2 {
              n4253 = property on="メイン測定ボタン_単発 3" class="Bool (指定)"("DisabledEnum"=w6888) -> ()  [unwired: 2 in, 2 out]
              n4254 = property on="メイン測定ボタン_連続 3" class="Bool (指定)"("DisabledEnum"=w6888) -> ()  [unwired: 2 in, 2 out]
            }
            frame 3 {
              n4255 = property on="メイン測定ボタン_単発 4" class="Bool (指定)"("DisabledEnum"=w6889) -> ()  [unwired: 2 in, 2 out]
            }
            frame 4 {
              n4256 = property on="メイン測定ボタン_単発 5" class="Bool (指定)"("DisabledEnum"=w6890) -> ()  [unwired: 2 in, 2 out]
              n4257 = property on="メイン測定ボタン_連続 5" class="Bool (指定)"("DisabledEnum"=w6890) -> ()  [unwired: 2 in, 2 out]
            }
            frame 5 {
              n4258 = property on="メイン測定ボタン_連続 6" class="Bool (指定)"("DisabledEnum"=w6891) -> ()  [unwired: 2 in, 2 out]
              n4259 = property on="メイン測定ボタン_単発 6" class="Bool (指定)"("DisabledEnum"=w6891) -> ()  [unwired: 2 in, 2 out]
            }
            frame 6 {
              n4260 = property on="メイン測定ボタン_連続 7" class="Bool (指定)"("DisabledEnum"=w6892) -> ()  [unwired: 2 in, 2 out]
              n4261 = property on="メイン測定ボタン_単発 7" class="Bool (指定)"("DisabledEnum"=w6892) -> ()  [unwired: 2 in, 2 out]
            }
            frame 7 {
              n4262 = property on="メイン測定ボタン_単発 8" class="Bool (指定)"("DisabledEnum"=w6893) -> ()  [unwired: 2 in, 2 out]
              n4263 = property on="メイン測定ボタン_連続 8" class="Bool (指定)"("DisabledEnum"=w6893) -> ()  [unwired: 2 in, 2 out]
            }
            frame 8 {
              n4264 = property on="メイン測定ボタン_単発 9" class="Bool (指定)"("DisabledEnum"=w6894) -> ()  [unwired: 2 in, 2 out]
              n4265 = property on="メイン測定ボタン_連続 9" class="Bool (指定)"("DisabledEnum"=w6894) -> ()  [unwired: 2 in, 2 out]
            }
            frame 9 {
              n4266 = property on="メイン測定ボタン_単発 10" class="Bool (指定)"("DisabledEnum"=w6895) -> ()  [unwired: 2 in, 2 out]
              n4267 = property on="メイン測定ボタン_連続 10" class="Bool (指定)"("DisabledEnum"=w6895) -> ()  [unwired: 2 in, 2 out]
            }
            frame 10 {
              n4268 = property on="メイン測定ボタン_単発 11" class="Bool (指定)"("DisabledEnum"=w6896) -> ()  [unwired: 2 in, 2 out]
              n4269 = property on="メイン測定ボタン_連続 11" class="Bool (指定)"("DisabledEnum"=w6896) -> ()  [unwired: 2 in, 2 out]
            }
            frame 11 {
              n4270 = property on="メイン測定ボタン_連続 12" class="Bool (指定)"("DisabledEnum"=w6897) -> ()  [unwired: 2 in, 2 out]
              n4271 = property on="メイン測定ボタン_単発 12" class="Bool (指定)"("DisabledEnum"=w6897) -> ()  [unwired: 2 in, 2 out]
            }
          }
        }
        n4272 = property on="TOPページへ" class="Bool"("DisabledEnum"=w6865) -> ()  [unwired: 2 in, 2 out]
        n4273 = property on="保存して終了" class="Bool"("DisabledEnum"=w6865) -> ()  [unwired: 2 in, 2 out]
        n4274 = property on="保存せずに" class="Bool"("DisabledEnum"=w6865) -> ()  [unwired: 2 in, 2 out]
      }
      event Value Change {
        w6898 = 12
        # "④ボタン操作時の他のボタン操作無効"
        # "※複製時\n①ブールボタン\n測定旧値\nが複製されているか確認\n②測定新値リセット用の作成\n対象の以外をリセットする\n③\nキュー\n④対象の連続ボタン以外複製する"
        # "③"
        # "旧値(ボタンが押される前と後)の値でグローバル_測定キャンセルボタンの\nTrue/Falseの切り替えを行う"
        # "②　例ケースが”メイン測定ボタン_連続2”の場合、\n測定新値リセット用2以外をリセットする"
        # "①"
        n4275 = event-data() -> ("OldVal"=w6900:T6)  [unwired: 1 in, 2 out]
        "測定旧値 5" <- w6900
        n4276 = Enqueue Element(queue=w6908, element="測定5", error in (no error)=w6905) -> (queue out=w6907:refnum<queue>, error out=w6906:errorcluster)  [unwired: 1 in, 1 out]
        n4277 = Select(t=TRUE, s=w6900, f=FALSE) -> (s? t:f=w6903:bool)
        n4278 = global write "測定キャンセルボタン.vi" "グローバル_測定キャンセルボタン"(w6903) -> ()
        n4279 = local write "G_メイン測定キャンセルボタン"(w6903) -> ()
        n4280 = for {
          N: w6898 -> [_]
          tunnel: FALSE -> [w6910]
          i -> [w6911]
          n4281 = case shown="4" w6911 {
            tunnel: w6910 -> [w6912 w6913 w6914 w6915 _ w6916 w6917 w6918 w6919 w6920 w6921 w6922]
            frame 0, Default {
              n4282 = local write "測定新値\nリセット用 1"(w6912) -> ()
            }
            frame 1 {
              n4283 = local write "測定新値\nリセット用 2"(w6913) -> ()
            }
            frame 2 {
              n4284 = local write "測定新値\nリセット用 3"(w6914) -> ()
            }
            frame 3 {
              n4285 = local write "測定新値\nリセット用 4"(w6915) -> ()
            }
            frame 4 {
            }
            frame 5 {
              n4286 = local write "測定新値\nリセット用 6"(w6916) -> ()
            }
            frame 6 {
              n4287 = local write "測定新値\nリセット用 7"(w6917) -> ()
            }
            frame 7 {
              n4288 = local write "測定新値\nリセット用 8"(w6918) -> ()
            }
            frame 8 {
              n4289 = local write "測定新値\nリセット用 9"(w6919) -> ()
            }
            frame 9 {
              n4290 = local write "測定新値\nリセット用 10"(w6920) -> ()
            }
            frame 10 {
              n4291 = local write "測定新値\nリセット用 11"(w6921) -> ()
            }
            frame 11 {
              n4292 = local write "測定新値\nリセット用 12"(w6922) -> ()
            }
          }
        }
        n4293 = for {
          N: w6898 -> [_]
          tunnel: w6904 -> [w6923]
          i -> [w6924]
          n4294 = case shown="11" w6924 {
            tunnel: w6923 -> [w6925 w6926 w6927 w6928 w6929 w6930 w6931 w6932 w6933 w6934 w6935 w6936]
            frame 0, Default {
              n4295 = property on="メイン測定ボタン_単発 1" class="Bool (指定)"("DisabledEnum"=w6925) -> ()  [unwired: 2 in, 2 out]
              n4296 = property on="メイン測定ボタン_連続 1" class="Bool (指定)"("DisabledEnum"=w6925) -> ()  [unwired: 2 in, 2 out]
            }
            frame 1 {
              n4297 = property on="メイン測定ボタン_単発 2" class="Bool (指定)"("DisabledEnum"=w6926) -> ()  [unwired: 2 in, 2 out]
              n4298 = property on="メイン測定ボタン_連続 2" class="Bool (指定)"("DisabledEnum"=w6926) -> ()  [unwired: 2 in, 2 out]
            }
            frame 2 {
              n4299 = property on="メイン測定ボタン_単発 3" class="Bool (指定)"("DisabledEnum"=w6927) -> ()  [unwired: 2 in, 2 out]
              n4300 = property on="メイン測定ボタン_連続 3" class="Bool (指定)"("DisabledEnum"=w6927) -> ()  [unwired: 2 in, 2 out]
            }
            frame 3 {
              n4301 = property on="メイン測定ボタン_単発 4" class="Bool (指定)"("DisabledEnum"=w6928) -> ()  [unwired: 2 in, 2 out]
              n4302 = property on="メイン測定ボタン_連続 4" class="Bool (指定)"("DisabledEnum"=w6928) -> ()  [unwired: 2 in, 2 out]
            }
            frame 4 {
              n4303 = property on="メイン測定ボタン_単発 5" class="Bool (指定)"("DisabledEnum"=w6929) -> ()  [unwired: 2 in, 2 out]
            }
            frame 5 {
              n4304 = property on="メイン測定ボタン_連続 6" class="Bool (指定)"("DisabledEnum"=w6930) -> ()  [unwired: 2 in, 2 out]
              n4305 = property on="メイン測定ボタン_単発 6" class="Bool (指定)"("DisabledEnum"=w6930) -> ()  [unwired: 2 in, 2 out]
            }
            frame 6 {
              n4306 = property on="メイン測定ボタン_連続 7" class="Bool (指定)"("DisabledEnum"=w6931) -> ()  [unwired: 2 in, 2 out]
              n4307 = property on="メイン測定ボタン_単発 7" class="Bool (指定)"("DisabledEnum"=w6931) -> ()  [unwired: 2 in, 2 out]
            }
            frame 7 {
              n4308 = property on="メイン測定ボタン_単発 8" class="Bool (指定)"("DisabledEnum"=w6932) -> ()  [unwired: 2 in, 2 out]
              n4309 = property on="メイン測定ボタン_連続 8" class="Bool (指定)"("DisabledEnum"=w6932) -> ()  [unwired: 2 in, 2 out]
            }
            frame 8 {
              n4310 = property on="メイン測定ボタン_単発 9" class="Bool (指定)"("DisabledEnum"=w6933) -> ()  [unwired: 2 in, 2 out]
              n4311 = property on="メイン測定ボタン_連続 9" class="Bool (指定)"("DisabledEnum"=w6933) -> ()  [unwired: 2 in, 2 out]
            }
            frame 9 {
              n4312 = property on="メイン測定ボタン_単発 10" class="Bool (指定)"("DisabledEnum"=w6934) -> ()  [unwired: 2 in, 2 out]
              n4313 = property on="メイン測定ボタン_連続 10" class="Bool (指定)"("DisabledEnum"=w6934) -> ()  [unwired: 2 in, 2 out]
            }
            frame 10 {
              n4314 = property on="メイン測定ボタン_単発 11" class="Bool (指定)"("DisabledEnum"=w6935) -> ()  [unwired: 2 in, 2 out]
              n4315 = property on="メイン測定ボタン_連続 11" class="Bool (指定)"("DisabledEnum"=w6935) -> ()  [unwired: 2 in, 2 out]
            }
            frame 11 {
              n4316 = property on="メイン測定ボタン_連続 12" class="Bool (指定)"("DisabledEnum"=w6936) -> ()  [unwired: 2 in, 2 out]
              n4317 = property on="メイン測定ボタン_単発 12" class="Bool (指定)"("DisabledEnum"=w6936) -> ()  [unwired: 2 in, 2 out]
            }
          }
        }
        n4318 = property on="TOPページへ" class="Bool"("DisabledEnum"=w6904) -> ()  [unwired: 2 in, 2 out]
        n4319 = property on="保存して終了" class="Bool"("DisabledEnum"=w6904) -> ()  [unwired: 2 in, 2 out]
        n4320 = property on="保存せずに" class="Bool"("DisabledEnum"=w6904) -> ()  [unwired: 2 in, 2 out]
      }
      event Value Change {
        w6937 = 12
        # "④ボタン操作時の他のボタン操作無効"
        # "※複製時\n①ブールボタン\n測定旧値\nが複製されているか確認\n②測定新値リセット用の作成\n対象の以外をリセットする\n③\nキュー\n④対象の連続ボタン以外複製する"
        # "③"
        # "旧値(ボタンが押される前と後)の値でグローバル_測定キャンセルボタンの\nTrue/Falseの切り替えを行う"
        # "②　例ケースが”メイン測定ボタン_連続2”の場合、\n測定新値リセット用2以外をリセットする"
        # "①"
        n4321 = event-data() -> ("OldVal"=w6939:T6)  [unwired: 1 in, 2 out]
        "測定旧値 6" <- w6939
        n4322 = Enqueue Element(queue=w6947, element="測定6", error in (no error)=w6944) -> (queue out=w6946:refnum<queue>, error out=w6945:errorcluster)  [unwired: 1 in, 1 out]
        n4323 = Select(t=TRUE, s=w6939, f=FALSE) -> (s? t:f=w6942:bool)
        n4324 = global write "測定キャンセルボタン.vi" "グローバル_測定キャンセルボタン"(w6942) -> ()
        n4325 = local write "G_メイン測定キャンセルボタン"(w6942) -> ()
